vi "Vision Research Phantom Series PhCon PhGetVideoFrNr.vi"(0 "CN in":u32=1, 5 "Error In (no error)":errorcluster) -> (14 "CN out":u32=1, 16 "pCrtIM":i32, 19 "Error Out":errorcluster)   [LabVIEW 2013, in "VRI.lvlib"]
doc: "PhCon.dll\n\nPhGetVideoFrNr\nHRESULT PhGetVideoFrNr(UINT CN, int* pCrtIm)\n\nParameters Description\nCN (in) Camera number.\npCrtIm (out) Pointer to the result: current image number played back\n to the video.\nReturn HRESULT (0 = Ok)\nComments Gets the frame number that is played back to the video\n out at this moment. It can be used to update a browse\n slider or a numeric display in a video player."
uses:
  VRI.lvlib
  Phantom DLLs/PhCon.Dll
panel:
  # "For instructions on the use of this VI, press Ctrl+H to display the help window and move the mouse over the icon, controls, and indicators"
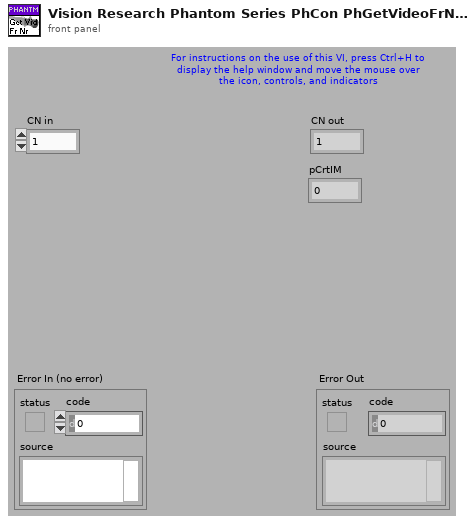
[diagram p1: front panel]
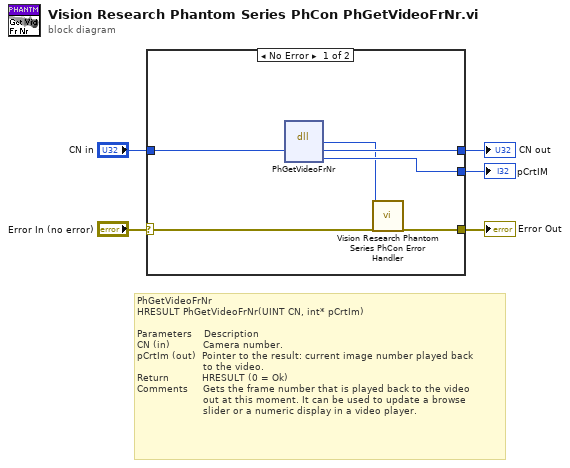
[diagram p0: block diagram]
diagram:
  # "PhGetVideoFrNr\nHRESULT PhGetVideoFrNr(UINT CN, int* pCrtIm)\n\nParameters    Description\nCN (in)           Camera number.\npCrtIm (out)  Pointer to the result: current image number played back\n                      to the video.\nReturn           HRESULT (0 = Ok)\nComments     Gets the frame number that is played back to the video\n                      out at this moment. It can be used to update a browse\n                      slider or a numeric display in a video player."
  n1 = case shown="No Error" "Error In (no error)" {
    selector: "Error In (no error)" -> [w11 w13]
    tunnel: [w10 w13] -> w4
    tunnel: "CN in" -> [w9 w12]
    tunnel: [w8 w12] -> w2
    tunnel: [w7 _] -> w1
    frame No Error {
      n2 = dll-call lib="C:/Projects/SDK/64-bit/Vision Research Phantom Series Labview Driver/Phantom DLLs/PhCon.dll" fn="PhGetVideoFrNr"("CN"=w9) -> ("HRESULT"=w6:i32, "CN"=w8:u32, "pCrtIm"=w7:i32)  [unwired: 3 in, 3 out]
      n3 = call "Vision Research Phantom Series PhCon Error Handler.vi"("ErrNo"=w6, "Error In (no error)"=w11) -> ("Error Out"=w10:errorcluster)  [unwired: 17 out]
    }
    frame Error {
    }
  }
  "Error Out" <- w4
  "CN out" <- w2
  "pCrtIM" <- w1
